vi "get paramater min max.vi"(8 "error in (no error)":errorcluster, 10 "parameter name":string, 11 "Simulated Camera in":refnum<class "Simulated Camera.lvclass">) -> (0 "error out":errorcluster, 1 "min":dbl, 2 "max":dbl, 3 "Simulated Camera out":refnum<class "Simulated Camera.lvclass">)   [LabVIEW 2018, in "Simulated Camera.lvclass"]
uses:
  Simulated Camera.lvclass
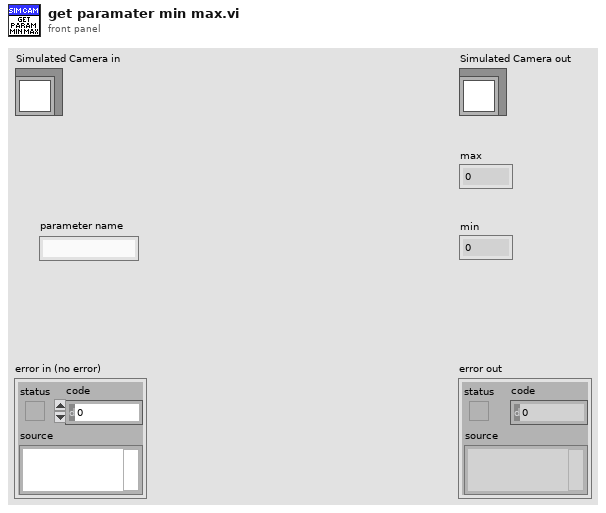
[diagram p1: front panel]
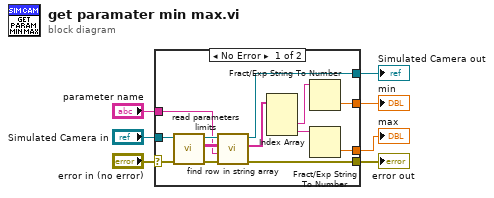
[diagram p0: block diagram]
diagram:
  n1 = case shown="No Error" "error in (no error)" {
    selector: "error in (no error)" -> [w15 w22]
    tunnel: [w10 w22] -> w6
    tunnel: [w8 w21] -> w4
    tunnel: "Simulated Camera in" -> [w14 w21]
    tunnel: [w12 _] -> w3
    tunnel: [w11 _] -> w2
    tunnel: "parameter name" -> [w9 _]
    frame No Error {
      n2 = call "read parameters limits.vi"("error in (no error)"=w15, "Simulated_CCD_Camera in"=w14) -> ("error out"=w13:errorcluster, "limit values spreadsheet"=w20:string[][], "Simulated_CCD_Camera out"=w19:refnum<class "Simulated Camera.lvclass">)  [unwired: 7 in]
      n3 = call "find row in string array.vi"("error in (no error)"=w13, "parameter name"=w9, "limit values"=w20, "Simulated_CCD_Camera in"=w19) -> ("error out"=w10:errorcluster, "row"=w18:string[], "Simulated_CCD_Camera out"=w8:refnum<class "Simulated Camera.lvclass">)  [unwired: 5 in]
      n4 = Index Array(array=w18) -> (element #2=w17:string, element #3=w16:string)  [unwired: 3 in, 1 out]
      n5 = Fract/Exp String To Number(string=w17) -> (number=w12:dbl)  [unwired: 3 in, 1 out]
      n6 = Fract/Exp String To Number(string=w16) -> (number=w11:dbl)  [unwired: 3 in, 1 out]
    }
    frame Error {
    }
  }
  "error out" <- w6
  "Simulated Camera out" <- w4
  "max" <- w2
  "min" <- w3
